vi "FL_Segment_map_by_color.vi"(2 "Array of presence count in":u32[][](array[numeric]), 3 "Array of the segment to color correspondences":u32[][](array[numeric]), 4 "Array of the pixel to color correspondences":u32[][](array[numeric]), 5 "Mouse abs. coordinates, pix":T1) -> (0 "Array of presence count out":u32[][](array[numeric]), 1 "Current segment' number":u32)   [LabVIEW 2018, in "Tracker.lvlib"]
uses:
  Tracker.lvlib
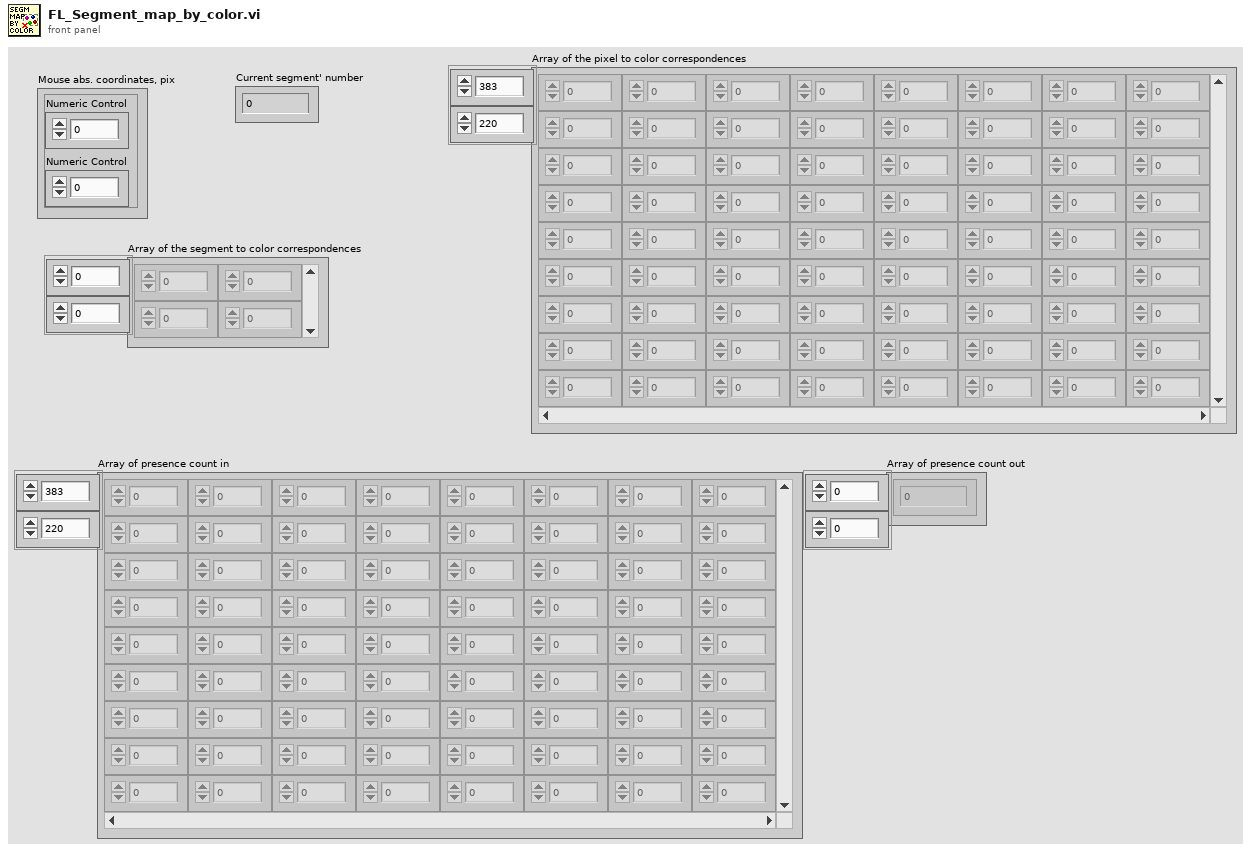
[diagram p1: front panel]
types:
  T1 = cluster{"Numeric Control":dbl, "Numeric Control":dbl}
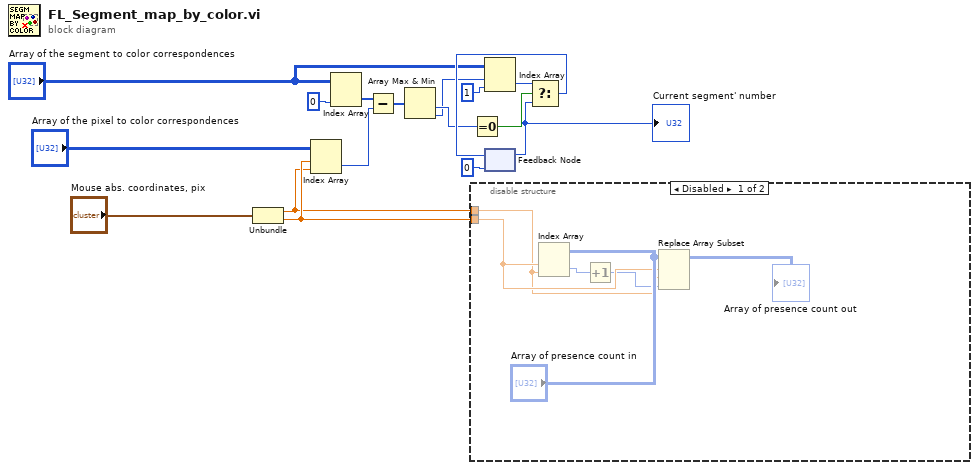
[diagram p0: block diagram]
diagram:
  n1 = Unbundle("Mouse abs. coordinates, pix") -> ("Numeric Control"=w1:dbl, "Numeric Control"=w2:dbl)
  n2 = Index Array(array="Array of the pixel to color correspondences", index (row)=w2, index (col)=w1) -> (element=w7:u32)
  n3 = Index Array(array="Array of the segment to color correspondences", index (col)=0 ("disabled index (col)")) -> (element=w6:u32[])  [unwired: 1 in]
  n4 = Subtract(x=w6, y=w7) -> (x-y=w8:u32[])
  n5 = Array Max & Min(array=w8) -> (min value=w12:u32, min index (indices)=w10:i32)  [unwired: 2 out]
  n6 = disable-structure shown="Disabled" {
    disable-tunnel: w2 -> [w22 _]
    disable-tunnel: w1 -> [w21 _]
    frame Disabled {
      n7 = Index Array(array="Array of presence count in", index (row)=w22, index (col)=w21) -> (element=w19:u32)
      n8 = Increment(x=w19) -> (x+1=w18:u32)
      n9 = Replace Array Subset(array="Array of presence count in", new element=w18, index (row)=w22, index (col)=w21) -> (→"Array of presence count out":u32[][])
    }
    frame Enabled {
    }
  }
  n10 = Equal To 0?(x=w12) -> (x = 0?=w14:bool)
  n11 = Index Array(array="Array of the segment to color correspondences", index (row)=w10, index (col)=1 ("disabled index (col)")) -> (element=w13:u32)
  n12 = feedback #1(u32 0 ("Color for central segment")) -> (w16:u32)
  "Current segment' number" <- w16
  n13 = Select(t=w13, s=w14, f=w16) -> (s? t:f=w15:u32)
  n14 = feedback-in #1(w15) -> ()
